vi "dac_update.vi"(3 "error in":errorcluster, 4 "Micron config":T1, 5 "DAC command":sgl[](array[numeric])) -> (0 "error out":errorcluster)   [LabVIEW 2010]
uses:
  initialization/micron_config.ctl
  <vilib>/DAQmx/write.llb/DAQmx Write (Analog 1D DBL NChan 1Samp).vi
  <vilib>/daqmx/miscellaneous.llb/DAQmx Fill In Error Info.vi
panel:
  in  "DAC range":sgl=5.0
  # "DAC range limit we enforce."
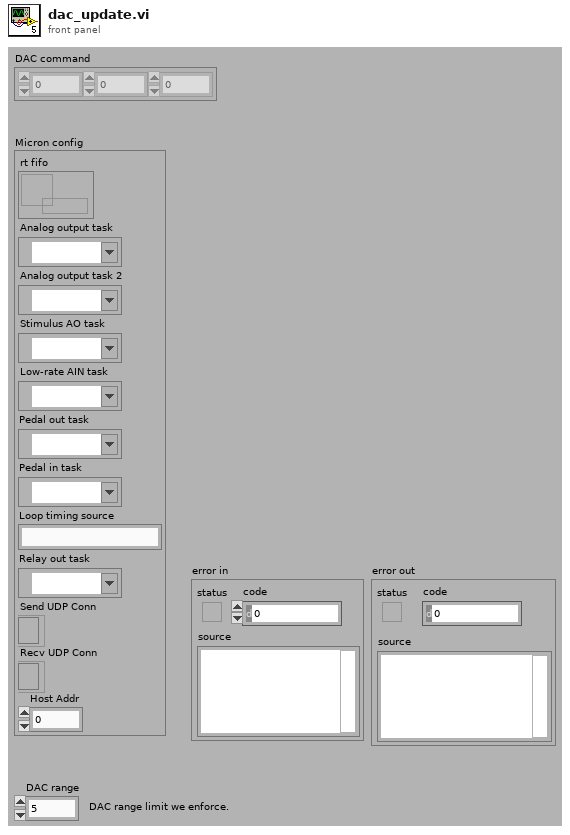
[diagram p1: front panel]
types:
  T1 = typedef "micron_config.ctl" = cluster{"rt fifo":refnum<k33>, "Analog output task":refnum<k21>, "Analog output task 2":refnum<k21>, "Stimulus AO task":refnum<k21>, "Low-rate AIN task":refnum<k21>, "Pedal out task":refnum<k21>, "Pedal in task":refnum<k21>, "Loop timing source":string, "Relay out task":refnum<k21>, "Send UDP Conn":refnum<k16>, "Recv UDP Conn":refnum<k16>, "Host Addr":dbl}
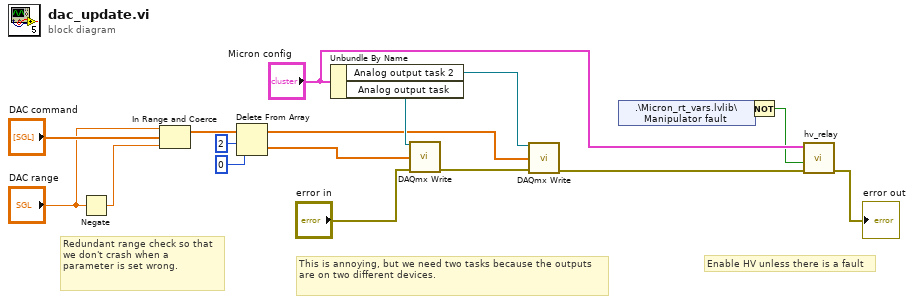
[diagram p0: block diagram]
diagram:
  # "Redundant range check so that we don't crash when a parameter is set wrong."
  # "Enable HV unless there is a fault"
  # "This is annoying, but we need two tasks because the outputs are on two different devices."
  n1 = Negate(x="DAC range") -> (-x=w3:sgl)
  n2 = In Range and Coerce(upper limit="DAC range", x="DAC command", lower limit=w3) -> (coerced(x)=w1:sgl[])  [unwired: 1 out]
  n3 = Delete From Array(array=w1, length=2, index=0) -> (deleted portion=w12:sgl[], array with subset deleted=w11:sgl[])
  n4 = Unbundle By Name("Micron config") -> ("Analog output task 2"=w14:refnum<k21>, "Analog output task"=w15:refnum<k21>)
  n5 = call-poly <vilib>:"DAQmx Write.vi"("task/channels in"=w15, "data"=w12, "error in"="error in") -> ("error out"=w16:errorcluster)  [unwired: 1 in, 11 out]
  n6 = call-poly <vilib>:"DAQmx Write.vi"("task/channels in"=w14, "data"=w11, "error in"=w16) -> ("error out"=w6:errorcluster)  [unwired: 1 in, 11 out]
  n7 = shared-variable ".\\Micron_rt_vars.lvlib\\Manipulator fault"() -> (w8:bool)  [unwired: 2 out]
  n8 = Not(x=w8) -> (.not. x?=w7:bool)
  n9 = call "hv_relay.vi"("error in"=w6, "data"=w7, "Micron config"="Micron config") -> ("error out"=→"error out":errorcluster)  [unwired: 8 out]
